vi "GenINI_Read_Template.vi"(8 "error in (no error)":errorcluster, 11 "INI path":path) -> (0 "error out":errorcluster, 3 "INI path out":path)   [LabVIEW 2009]
uses:
  <vilib>/Utility/config.llb/NI_LVConfig.lvlib
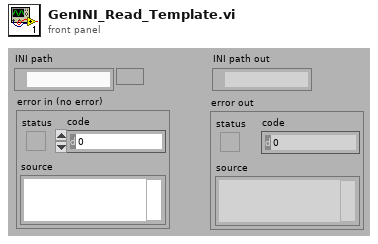
[diagram p1: front panel]
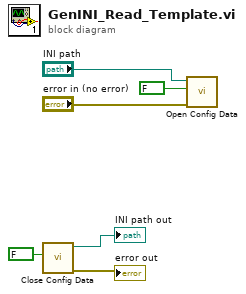
[diagram p0: block diagram]
diagram:
  n1 = call <vilib>:"Close Config Data.vi"("write file if changed (T)"=FALSE) -> ("error out"=→"error out":errorcluster, "file path"=→"INI path out":path)  [unwired: 9 in]
  n2 = call <vilib>:"Open Config Data.vi"("error in (no error)"="error in (no error)", "create file if necessary (T)"=FALSE, "configuration file path"="INI path") -> ()  [unwired: 6 in, 3 out]
